vi "Do.vi"(8 "error in (no error)":errorcluster, 10 "Actor in":refnum<class "Actor.lvclass">, 11 "New Message Msg":refnum<class "New Message Msg.lvclass">) -> (0 "error out":errorcluster, 2 "Actor out":refnum<class "Actor.lvclass">)   [LabVIEW 2017, in "BuildWorker.lvlib" / "New Message Msg.lvclass"]
doc: "This VI delivers the message to the actor by calling the appropriate method(s) on the actor."
uses:
  New Message Msg.lvclass
  C:/Users/Public/Documents/wc/BuildFarm/src/LabVIEW/vi.lib/BenjaminR/Build Farm/Actors/Communication/WebSocket Client/WebSocket Client Messages/New Message Msg/New Message Msg.lvclass
  <vilib>/ActorFramework/Actor/Actor.lvclass
  BuildWorker/BuildWorker.lvclass
  C:/Program Files (x86)/National Instruments/LabVIEW 2017/vi.lib/ActorFramework/Actor/Actor.lvclass
  Communication/WebSocket Client/WebSocket Client Messages/New Message Msg/New Message Msg.lvclass/New Message Msg.ctl
  Communication/WebSocket Client/WebSocket Client Messages/New Message Msg/New Message Msg.lvclass
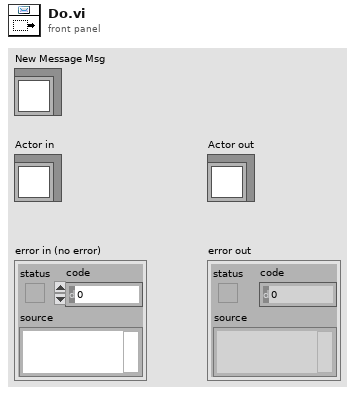
[diagram p1: front panel]
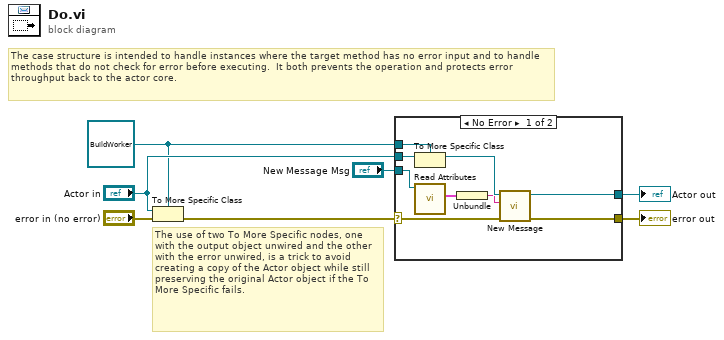
[diagram p0: block diagram]
diagram:
  w2 = refnum<class "BuildWorker.lvclass"> refnum ("Actor in")
  # "The use of two To More Specific nodes, one with the output object unwired and the other with the error unwired, is a trick to avoid creating a copy of the Actor object while still preserving the original Actor object if the To More Specific fails."
  # "The case structure is intended to handle instances where the target method has no error input and to handle methods that do not check for error before executing.  It both prevents the operation and protects error throughput back to the actor core."
  n1 = To More Specific Class(target class=w2, reference="Actor in", error in="error in (no error)") -> (error out=w6:errorcluster)  [unwired: 1 out]
  n2 = case shown="No Error" w6 {
    selector: w6 -> [w14 w18]
    tunnel: [w16 w18] -> w5
    tunnel: [w15 w17] -> w4
    tunnel: "Actor in" -> [w13 w17]
    tunnel: w2 -> [w12 _]
    tunnel: "New Message Msg" -> [w9 _]
    frame No Error {
      n3 = To More Specific Class(target class=w12, reference=w13) -> (specific class reference=w11:refnum<class "BuildWorker.lvclass">)  [unwired: 1 in, 1 out]
      n4 = call "Read Attributes.vi"("New Message Msg"=w9) -> ("Payload"=w10:cluster{"New Message":string})  [unwired: 10 in]
      n5 = Unbundle(w10) -> ("New Message"=w8:string)
      n6 = call "New Message.vi"("error in (no error)"=w14, "New Message"=w8, "BuildWorker in"=w11) -> ("error out"=w16:errorcluster, "BuildWorker out"=w15:refnum<class "BuildWorker.lvclass">)  [unwired: 7 in]
    }
    frame Error {
      # "If type check fails, pass the original object out again."
    }
  }
  "error out" <- w5
  "Actor out" <- w4
